vi "UART.vi"() -> ()   [LabVIEW 2019]
uses:
  <vilib>/myRIO/Instrument Drivers/Onboard IO/UART/typedef/VISA Configuration.ctl
  <vilib>/userdefined/High Color/nirio_resource_hc.ctl
  <vilib>/Utility/error.llb/Error Cluster From Error Code.vi
  <vilib>/myRIO/Common/Instrument Driver Framework/ELVIS III v1.0/ELVIS III v1.1 Open.vi
  <vilib>/myRIO/Common/Instrument Driver Framework/ELVIS III v1.0/Resource Manager/vis/ELVIS III v1.0 Reserve Channel List.vi
  <vilib>/myRIO/Common/Instrument Driver Framework/myRIO v1.0/myRIO v1.0 Close.vi
  <vilib>/Instr/_visa.llb/VISA Configure Serial Port (Instr).vi
  <vilib>/myRIO/Common/Instrument Driver Framework/Utilities/vis/FPGA Ref Manager.vi
  <vilib>/myRIO/Common/Instrument Driver Framework/ELVIS III v1.0/ELVIS III v1.0 Reset FPGA.vi
  <vilib>/myRIO/Common/Instrument Driver Framework/myRIO v1.0/IRQ/vis/myRIO v1.0 IRQ Info FGV.vi
  <vilib>/myRIO/Common/Instrument Driver Framework/myRIO v1.0/IRQ/vis/myRIO v1.0 Timer IRQ Info FGV.vi
  <vilib>/myRIO/Common/Instrument Driver Framework/myRIO v1.0/IRQ/vis/myRIO v1.0 ISR Agent.vi
  <vilib>/myRIO/Instrument Drivers/Utilities/vis/Reset Index.vi
  <vilib>/myRIO/Common/Instrument Driver Framework/myRIO v1.0/Resource Manager/vis/myRIO v1.0 Block Write Resource Manager.vi
  <vilib>/myRIO/Express VI/Onboard IO/UART/UART Express VI.xnode
  <vilib>/myRIO/Instrument Drivers/Utilities/Utilities.lvlib
  <vilib>/myRIO/Instrument Drivers/Onboard IO/UART/UART.lvlib
  <vilib>/myRIO/Common/Instrument Driver Framework/Utilities/vis/Set_Get Target Info.vi
panel:
  out "Characters Read":string
  out "Character Count":u32
  in  "Characters to Write":string="Example string."
  # "ELVIS III Control IO"
  # "UART"
  # "Overview: Performs a loopback test on the Bank A UART lines (RX: A/DIO16, TX: A/DIO17).\nInstructions:\n1. Connect a wire from A/DIO16 to A/DIO17.\n2. Change the text within the Characters to Write.\n3. Run the VI.\n4. Notice Characters Read contains the same characters written to Characters to Write."
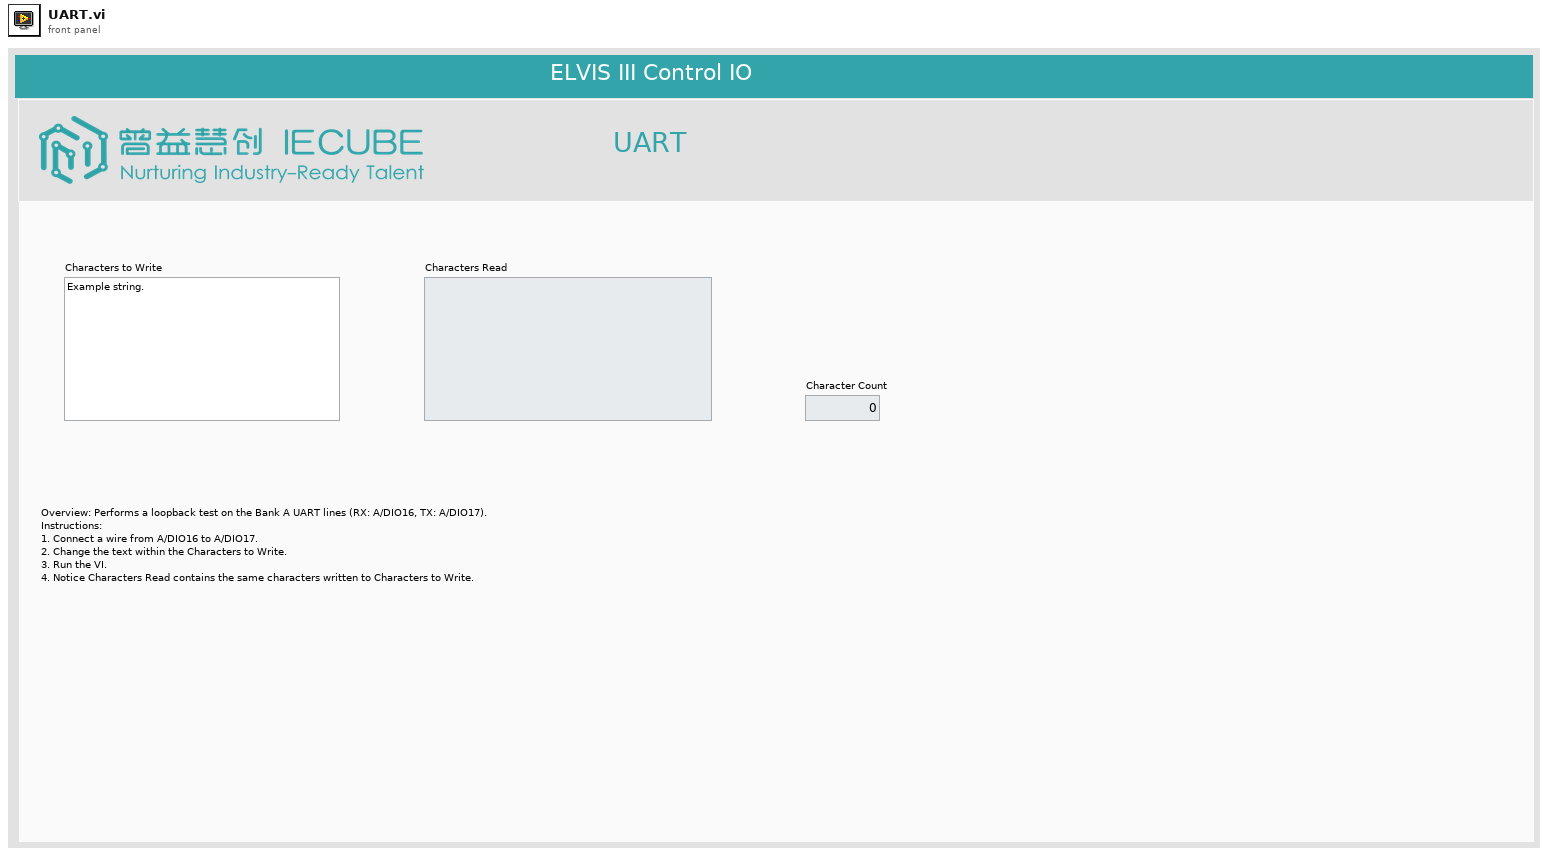
[diagram p1: front panel]
types:
  T1 = typedef "UART.lvlib/VISA Configuration.ctl" = cluster{"baud rate (9600)":u32, "data bits (8)":u16, "parity (0:none)":enum16{"None", "Odd", "Even", "Mark", "Space"}, "stop bits (10: 1 bit)":u16, "flow control (0:none)":u16, "termination char\n(0xA = '\\n' = LF) ":u8, "Enable Termination\nChar (T)":bool, "timeout (10sec)":u32}
  T2 = typedef "nirio_resource_hc.ctl" = tag
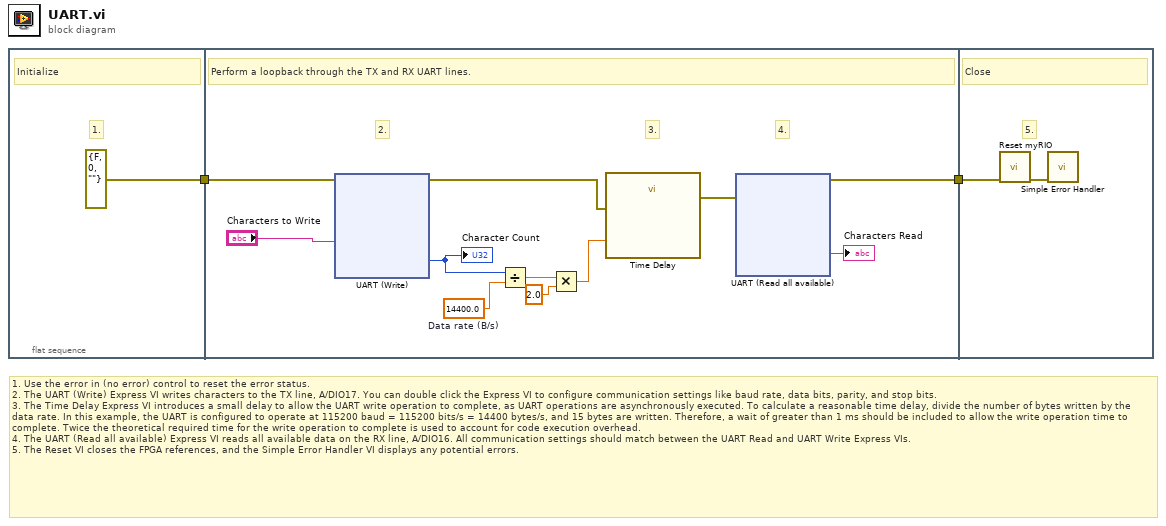
[diagram p0: block diagram]
diagram:
  # "1. Use the error in (no error) control to reset the error status.\n2. The UART (Write) Express VI writes characters to the TX line, A/DIO17. You can double click the Express VI to configure communication settings like baud rate, data bits, parity, and stop bits.\n3. The Time Delay Express VI introduces a small delay to allow the UART write operation to complete, as UART operations are asynchronously executed. To calculate a reasonable time delay, divide the number of bytes written by the data rate. In this example, the UART is configured to operate at 115200 baud = 115200 bits/s = 14400 bytes/s, and 15 bytes are written. Therefore, a wait of greater than 1 ms should be included to allow the write operation time to complete. Twice the theoretical required time for the write operation to complete is used to account for code execution overhead.\n4. The UART (Read all available) Express VI reads all available data on the RX line, A/DIO16. All communication settings should match between the UART Read and UART Write Express VIs.\n5. The Reset VI closes the FPGA references, and the Simple Error Handler VI displays any potential errors."
  n1 = flat-sequence {
    tunnel: [errorcluster {"status"=FALSE, "code"=0, "source"=""} ("Error In")] -> w1
    tunnel: [w14] -> w2
    tunnel: w1 -> [w13]
    tunnel: w2 -> [w105]
    frame #0 {
      # "1."
      # "Initialize"
    }
    frame #1 {
      w6 = 14400.0  # Data rate (B/s)
      # "4."
      # "3."
      # "2."
      # "Perform a loopback through the TX and RX UART lines."
      n2 = xnode "UART (Write)"("Characters to Write"="Characters to Write", "error in (no error)"=w13) -> ("Character Count"=w7:u32, "error out"=w11:errorcluster)
      "Character Count" <- w7
      n3 = Divide(x=w7, y=w6) -> (x/y=w8:dbl)
      n4 = Multiply(x=w8, y=2.0) -> (x*y=w4:dbl)
      n5 = call "Time Delay"("error in (no error)"=w11, "Delay Time (s)"=w4) -> ("error out"=w10:errorcluster)  [unwired: 9 in]
      n6 = xnode "UART (Read all available)"("error in (no error)"=w10) -> ("Characters Read"=→"Characters Read":string, "error out"=w14:errorcluster)
    }
    frame #2 {
      # "5."
      # "Close"
      n7 = call <vilib>:"Reset myRIO.vi"("error in (no error)"=w105) -> ("error out"=w104:errorcluster)  [unwired: 10 in]
      n8 = call <vilib>:"Simple Error Handler.vi"("error in (no error)"=w104) -> ()  [unwired: 4 in, 5 out]
    }
  }
